vi "Version_Parse.vi"(0 "All_ERD_Data_Bundled_Brass in":T2, 5 "Converted Data Out":T1 {"CRC" format="%04x"; "Length" format="%02x"; "Command" format="%02x"; "Destination" format="%02x"; "Source" format="%02x"}, 11 "Error In":errorcluster) -> (4 "All_ERD_Data_Bundled_Brass out":T2, 15 "Error Out":errorcluster)   [LabVIEW 2021]
uses:
  type defs/All_Bundled_Data.ctl
  type defs/Version.ctl
  type defs/ERD_Always_Show.ctl
  type defs/Brass Matrix.ctl
  type defs/CSV_File_String_Arrays.ctl
  type defs/Redundant.ctl
  type defs/Algorithms.ctl
  type defs/ATC_Data.ctl
  type defs/Fault Table Array.ctl
  type defs/Fault_Table_Info.ctl
  Dryer Tool (Commercial 2)/JL Dryer Tool Support/type defs/ERD_RJ45.ctl
  Dryer Tool (Commercial 2)/JL Dryer Tool Support/type defs/ERD_Commercial_Laundry.ctl
  type defs/BootloaderVersion.ctl
  Common/LabVIEW GEA2 Toolkit/GEA3/type defs/Data Out.ctl
panel:
  # "Wet Load Size"
  # "Dry Load Size"
  # "OOB"
  # "Wet Load Size"
  # "Dry Load Size"
  # "OOB"
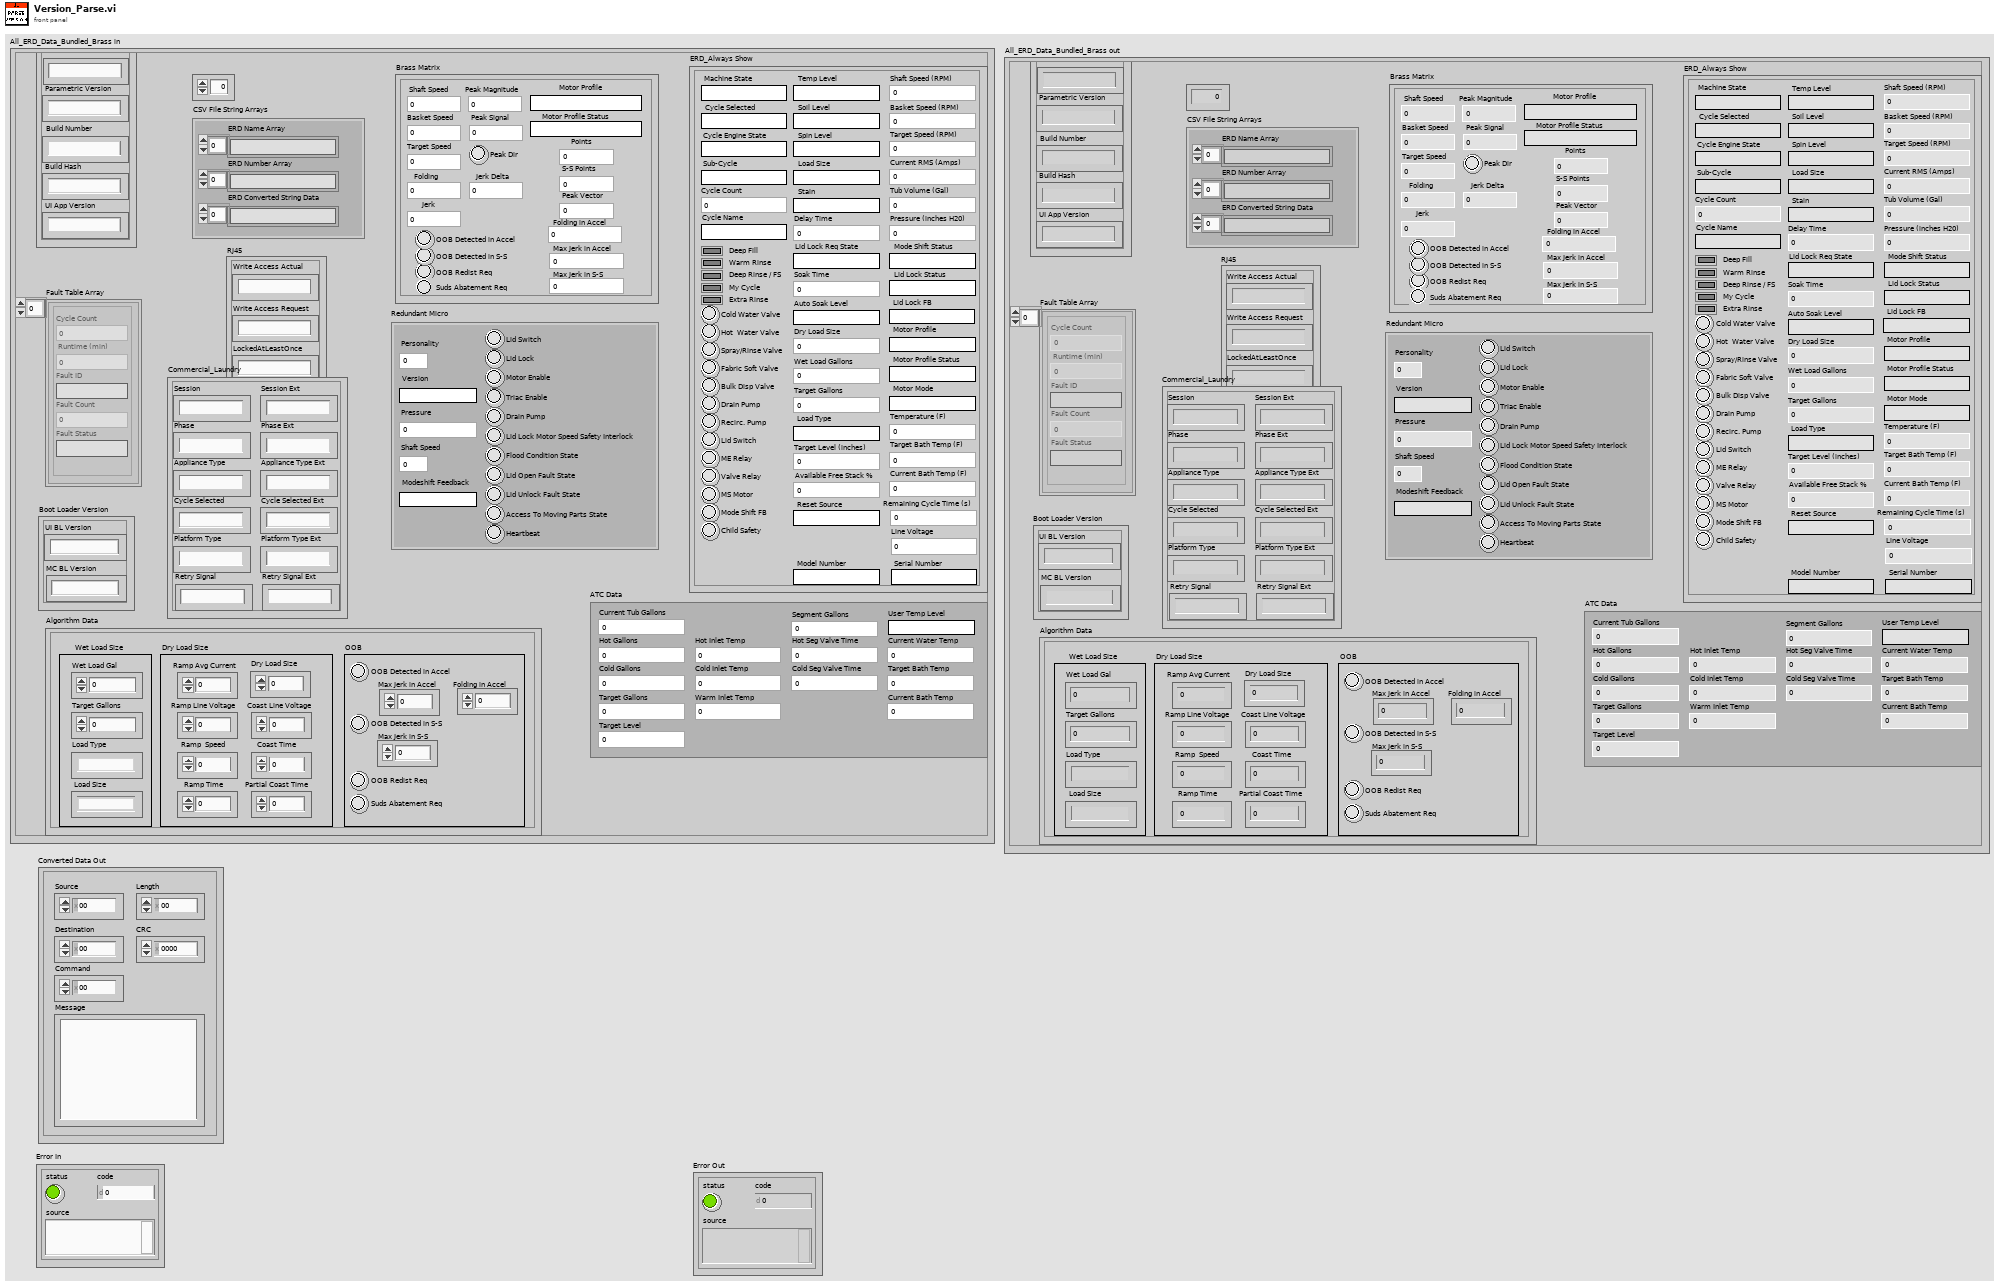
[diagram p1: front panel]
types:
  T1 = typedef "Data Out.ctl" = cluster{"Source":u8, "Destination":u8, "Command":u8, "Length":u8, "CRC":u16, "Message":string}
  T2 = typedef "All_Bundled_Data.ctl" = cluster{"Software MC":T3, "ERD_Always Show":T4, "Personality Set":u8, "Brass Matrix":T5, "CSV File String Arrays":T6, "Redundant Micro":T7, "Algorithm Data":T8, "ATC Data":T9, "Fault Table Array ":T10, "RJ45":T12, "Commercial_Laundry":T13, "Boot Loader Version":T14}
  T3 = typedef "Version.ctl" = cluster{"Build Number":string, "Build Hash ":string, "Application Version":string, "Parametric Version":string, "UI App Version":string}
  T4 = typedef "ERD_Always_Show.ctl" = cluster{"Basket Speed (RPM)":u16, "Machine State":string, "Tub Volume (Gal)":dbl, "Pressure (inches H20)":dbl, "Lid Switch ":bool, "Current RMS (Amps)":dbl, "Cycle Selected":string, "Lid Lock Status":string, "Mode Shift Status":string, "Spray/Rinse Valve":bool, "Fabric Soft Valve":bool, "Drain Pump":bool, "Recirc. Pump":bool, "Cycle Engine State":string, "Hot  Water Valve":bool, "Cold Water Valve":bool, "Motor Profile":string, "Motor Profile Status":string, "Motor Mode":string, "ME Relay":bool, "Cycle Count":u32, "Deep Rinse / FS":bool, "My Cycle":bool, "Soil Level":string, "Spin Level":string, "Stain":string, "Temp Level":string, "Load Size":string, "Delay Time":u16, "Soak Time":u16, "Deep Fill":bool, "Warm Rinse":bool, "Auto Soak Level":string, "Extra Rinse":bool, "Wet Load Gallons":dbl, "Target Gallons":dbl, "Sub-Cycle":string, "Load Type":string, "Target Level (inches)":dbl, "Valve Relay":bool, "Dry Load Size":dbl, "Shaft Speed (RPM) ":u16, "MS Motor":bool, "Mode Shift FB":bool, "Target Bath Temp (F)":dbl, "Temperature (F)":dbl, "Current Bath Temp (F)":dbl, "Lid Lock FB":string, "Lid Lock Req State":string, "Remaining Cycle Time (s)":u32, "Available Free Stack %":u8, "Child Safety":bool, "Target Speed (RPM)":u16, "Reset Source":string, "Line Voltage":dbl, "Cycle Name":string, "Bulk Disp Valve":bool, "Model Number":string, "Serial Number":string}
  T5 = typedef "Brass Matrix.ctl" = cluster{"Shaft Speed":u16, "Folding":i32, "Jerk":i32, "Basket Speed":u16, "Target Speed":u16, "Peak Signal":u8, " Peak Magnitude":dbl, "Folding in Accel":i32, "Max Jerk in Accel":i32, "Max Jerk in S-S":i32, "Motor Profile Status":string, "Motor Profile":string, "OOB Redist Req":bool, "OOB Detected in S-S":bool, "OOB Detected in Accel":bool, "Suds Abatement Req ":bool, "Peak Dir":bool, "Peak Vector":dbl, "S-S Points":u8, "Points":u8, "Jerk Delta":i32}
  T6 = typedef "CSV_File_String_Arrays.ctl" = cluster{"ERD Number Array":string[], "ERD Name Array":string[], "ERD Converted String Data":string[]}
  T7 = typedef "Redundant.ctl" = cluster{"Version":string, "Personality":u8, "Pressure ":dbl, "Shaft Speed":u16, "Modeshift Feedback":string, "Lid Switch":bool, "Lid Lock":bool, "Triac Enable":bool, "Drain Pump":bool, "Lid Lock Motor Speed Safety Interlock":bool, "Flood Condition State":bool, "Lid Open Fault State":bool, "Access To Moving Parts State":bool, "Heartbeat":bool, "Motor Enable":bool, "Lid Unlock Fault State":bool}
  T8 = typedef "Algorithms.ctl" = cluster{"Wet Load Gal":dbl, "Target Gallons":dbl, "Load Type":string, "Load Size":string, "Coast Time":u16, "Ramp Time":u16, "Ramp  Speed":u16, "Ramp Avg Current":dbl, "OOB Redist Req":bool, "OOB Detected in S-S":bool, "Folding in Accel":i32, "Max Jerk in Accel":i32, "Max Jerk in S-S":i32, "OOB Detected in Accel":bool, "Partial Coast Time":u16, "Dry Load Size":dbl, "Ramp Line Voltage ":dbl, "Coast Line Voltage":dbl, "Suds Abatement Req ":bool}
  T9 = typedef "ATC_Data.ctl" = cluster{"Current Tub Gallons":dbl, "Hot Gallons":dbl, "Cold Gallons":dbl, "Target Gallons":dbl, "Current Water Temp":dbl, "Target Level":dbl, "Target Bath Temp":dbl, "Current Bath Temp ":dbl, "Cold Inlet Temp":dbl, "Hot Inlet Temp":dbl, "Warm Inlet Temp":dbl, "Hot Seg Valve Time":u16, "Cold Seg Valve Time ":u16, "User Temp Level":string, "Segment Gallons":dbl}
  T10 = typedef "Fault Table Array.ctl" = T11[]
  T11 = typedef "Fault_Table_Info.ctl" = cluster{"Cycle Count":u32, " Runtime (min) ":u32, "Fault Status":string, "Fault ID":string, "Fault Count":u16}
  T12 = typedef "ERD_RJ45.ctl" = cluster{"Write Access Actual":string, "Write Access Request":string, "LockedAtLeastOnce":string}
  T13 = typedef "ERD_Commercial_Laundry.ctl" = cluster{"Session":string, "Phase":string, "Appliance Type":string, "Cycle Selected":string, "Platform Type":string, "Retry Signal":string, "Session Ext":string, "Phase Ext":string, "Appliance Type Ext":string, "Cycle Selected Ext":string, "Platform Type Ext":string, "Retry Signal Ext":string}
  T14 = typedef "BootloaderVersion.ctl" = cluster{"UI BL Version":string, "MC BL Version":string}
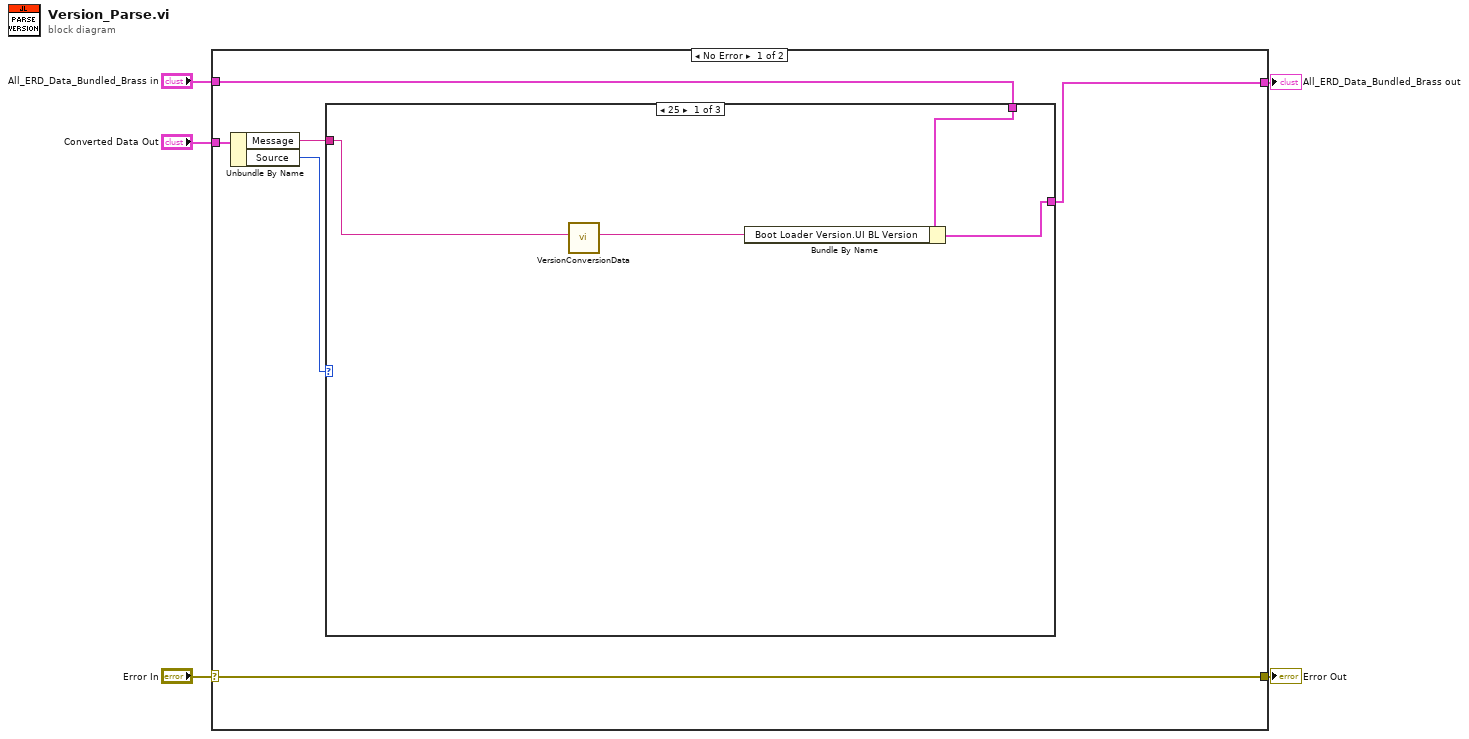
[diagram p0: block diagram]
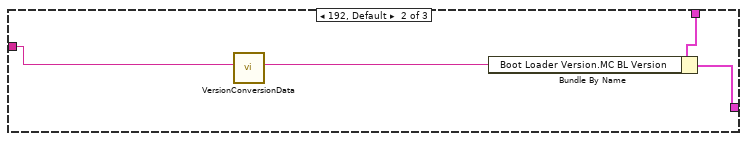
[diagram p2: hidden frame]
diagram:
  n1 = case shown="No Error" "Error In" {
    selector: "Error In" -> [w9 w22]
    tunnel: [w11 w21] -> w5
    tunnel: "All_ERD_Data_Bundled_Brass in" -> [w10 w21]
    tunnel: "Converted Data Out" -> [w8 _]
    tunnel: [w9 w22] -> w1
    frame No Error {
      n2 = Unbundle By Name(w8) -> ("Message"=w7:string, "Source"=w6:u8)
      n3 = case shown="25" w6 {
        tunnel: [w15 w19 w20] -> w11
        tunnel: w10 -> [w14 w18 w20]
        tunnel: w7 -> [w13 w16 _]
        frame 37 {
          n4 = call "VersionConversionData.vi"("Version In"=w13) -> ("Version Out"=w12:string)  [unwired: 9 in, 1 out]
          n5 = Bundle By Name(cluster=w14, "Boot Loader Version.UI BL Version"=w12) -> (w15:T2)
        }
        frame 192, Default {
          n6 = call "VersionConversionData.vi"("Version In"=w16) -> ("Version Out"=w17:string)  [unwired: 9 in, 1 out]
          n7 = Bundle By Name(cluster=w18, "Boot Loader Version.MC BL Version"=w17) -> (w19:T2)
        }
        frame 36 {
        }
      }
    }
    frame Error {
    }
  }
  "All_ERD_Data_Bundled_Brass out" <- w5
  "Error Out" <- w1
